vi "SR830 - Kepco - Hysteresis Measurment - Stepped DC.vi"() -> ()   [LabVIEW 2016]
uses:
  <vilib>/express/express shared/transition.llb/Dynamic To Waveform Array.vi
  <vilib>/express/express signal manip/GetorSetDDTAttributes/Set DDT Attributes/SetT0.vi
  <vilib>/express/express shared/transition.llb/Waveform Array To Dynamic.vi
  <vilib>/express/express signal manip/GetorSetDDTAttributes/Set DDT Attributes/Set DDT Properties.xnode
panel:
  out "Sample VDC (V)":dbl
  out "Over Temp":bool
  in  "Zero Field Wait Time (s)":u32=30
  out "Setup Data":T1
  in  "Sample Name":string="test"
  in  "Directory":string="D:\\JDark\\MTJ Cryostat\\test"
  out "Filename Out":path=path "D:/JDark/MTJ Cryostat/test/test-20mT-hysteresis.lvm"
  in  "Accepted Setup":bool
  in  "Verified Setup":bool
  out "Field Vs Res Noise":cluster{dbl[], dbl[]}(graph)={[-0.0544, 0.4456, 0.9352, 1.4248, 1.9143999999999999, 2.404, 2.8935999999999997, 3.3832, 3.8728, 4.362399999999999, 4.852, 5.3416, 5.8312, 6.320799999999999, 6.8104000000000005, 7.3, 7.7896, 8.2792, 8.768799999999999, 9.2584, 10.248000000000001, 10.7272, 11.216800000000001, 11.706399999999999, 12.196, 12.685599999999999, 13.1752, 13.6648, 14.154399999999999, 14.644, 15.133600000000001, 15.6232, 16.1128, 16.6024, 17.092, 17.581599999999998, 18.0712, 18.5608, 19.0504, 19.54, 20.0296, 19.519199999999998, 19.0296, 18.54, 18.0504, 17.5608, 17.0712, 16.581599999999998, 16.092, 15.6024, 15.112799999999998, 14.6232, 14.133600000000001, 13.644, 13.154399999999999, 12.6648, 12.1752, 11.685599999999999, 11.196, 10.706399999999999, 10.216800000000001, 9.7272, 9.237599999999999, 8.748000000000001, 7.7584, 7.2791999999999994, 6.7896, 6.3, 5.8104000000000005, 5.320799999999999, 4.8312, 4.3416, 3.8520000000000003, 3.3623999999999996, 2.8728, 2.3832, 1.8935999999999997, 1.4040000000000001, 0.9143999999999999, 0.42480000000000007, -0.06480000000000002, -0.5544, -1.044, -1.5335999999999999, -2.0232, -2.5128, -3.0023999999999997, -3.492, -3.9816, -4.4712, -4.9608, -5.4504, -5.94, -6.4296, -6.919199999999999, -7.4088, -7.8984000000000005, -8.387999999999998, -8.8776, -9.3672, -9.8568, -10.3464, -10.836, -11.3256, -11.815199999999999, -12.3048, -12.7944, -13.283999999999999, -13.7736, -14.2632, -14.7528, -15.7424, -16.2216, -16.711199999999998, -17.2008, -17.6904, -18.18, -18.6696, -19.159200000000002, -19.648799999999998, -20.138399999999997, -19.628, -19.138399999999997, -18.648799999999998, -18.159200000000002, -17.6696, -17.18, -16.6904, -16.2008, -15.711199999999998, -15.221599999999999, -14.732000000000001, -14.2424, -13.2528, -12.7736, -12.283999999999999, -11.7944, -11.3048, -10.815199999999999, -10.3256, -9.836, -9.3464, -8.8568, -8.3672, -7.877599999999999, -7.387999999999999, -6.8984000000000005, -6.4088, -5.919199999999999, -5.4296, -4.94, -4.4504, -3.9608, -3.4711999999999996, -2.9816, -2.492, -2.0023999999999997, -1.5128, -1.0231999999999999, -0.5335999999999999, -0.04400000000000004], [15446.997899211381, 33956.24923800761, 28583.62141204098, 32537.69937438095, 21226.11553919723, 21221.33942488045, 39173.4048903721, 26230.601252371347, 25250.361708040735, 35822.515248200485, 37581.515773031526, 23883.174686296858, 39995.65587105874, 17569.924451207833, 34863.32464679369, 18416.192176577308, 23302.25342512084, 32855.534688062005, 48354.66753159789, 26888.48894404787, 27946.841353229545, 28447.25655247211, 22692.535929595357, 30888.946076662316, 42324.47121995423, 35843.85501529699, 36799.549654445036, 33329.48011847423, 22851.300082707552, 41191.92793475303, 34456.720236005174, 26058.631203020544, 44746.53461020991, 37224.99718726645, 68825.00201996259, 42958.99230679308, 40714.67079910066, 57747.71988536508, 29691.254129653025, 64211.258772769135, 19160.606846375562, 46321.221303721766, 71029.59431320045, 46892.27695542654, 44799.75730671692, 66819.48067982277, 33651.5376743769, 59810.240340936194, 40119.21014462293, 32334.725091976245, 28529.285706498602, 23730.97499127908, 57610.91864749145, 22435.444676456966, 40951.30401185154, 25070.447710137123, 41949.69263686712, 45718.11923108557, 65627.3156788876, 56953.651543237196, 32173.835671959445, 52671.5915678221, 19668.458783462793, 66303.20158982599, 29710.854540049048, 31775.497941348356, 40549.964623149535, 51075.99354753492, 30654.539201948188, 39128.479352554976, 76442.95433228796, 39447.51980352633, 50016.20330851342, 31887.563882788363, 51028.591960972844, 10819.279889052948, 33818.527611194106, 28613.771934449134, 26922.398338747033, 48873.51208949818, 15542.950456565659, 36990.502142052654, 43527.933077723064, 44359.638776024505, 57036.44671814811, 39849.33042216752, 41185.472573773004, 39269.88832369224, 38812.156278821516, 34044.05435458031, 46110.809967419984, 26920.93030568665, 20022.36039942582, 30293.79168452148, 36986.91194556142, 31863.995532675028, 48564.8883204678, 31712.338377027238, 27426.89264464971, 30851.999129154938, 48273.56430512302, 29150.41172792822, 24567.903850798903, 63596.70014848106, 48763.27199117811, 37803.08487296523, 25487.82251127746, 36390.95236019352, 40160.54536019719, 34535.106643400075, 21909.398015546907, 27598.43480264338, 35167.06869216419, 21013.991394512836, 34624.77760643399, 30213.396643427317, 37149.78361918999, 43845.320556022314, 42048.2311943678, 27051.29365915422, 64603.25813602039, 43018.44966767505, 55993.00123154771, 50035.68025960878, 39493.42322008669, 32009.408479252674, 26595.55919730376, 42173.5517388975, 12637.40264403457, 39752.76755871613, 63107.71184796988, 40876.126484711815, 20174.17913949147, 42100.458189798745, 40400.4870213476, 24357.325777515885, 31546.25760360981, 54921.53998993925, 23599.30892344478, 34629.83814368073, 29691.38924623618, 41182.45982586981, 37153.31598804947, 14587.365677128682, 41348.93298571064, 10205.174478406218, 44091.93656368952, 31245.442862556854, 43901.36431959185, 32472.003090461087, 69163.31002984302, 21452.1832368206, 22799.206544846253, 35507.71909151544, 49297.22538812266, 29873.140517007283, 32041.329961389703, 53622.65124570277, 26624.64715323181, 29899.602878098507, 50511.70265602952]}
  out "TMR":cluster{dbl[], dbl[]}(graph)={[-0.0544, 0.4456, 0.9352, 1.4248, 1.9143999999999999, 2.404, 2.8935999999999997, 3.3832, 3.8728, 4.362399999999999, 4.852, 5.3416, 5.8312, 6.320799999999999, 6.8104000000000005, 7.3, 7.7896, 8.2792, 8.768799999999999, 9.2584, 10.248000000000001, 10.7272, 11.216800000000001, 11.706399999999999, 12.196, 12.685599999999999, 13.1752, 13.6648, 14.154399999999999, 14.644, 15.133600000000001, 15.6232, 16.1128, 16.6024, 17.092, 17.581599999999998, 18.0712, 18.5608, 19.0504, 19.54, 20.0296, 19.519199999999998, 19.0296, 18.54, 18.0504, 17.5608, 17.0712, 16.581599999999998, 16.092, 15.6024, 15.112799999999998, 14.6232, 14.133600000000001, 13.644, 13.154399999999999, 12.6648, 12.1752, 11.685599999999999, 11.196, 10.706399999999999, 10.216800000000001, 9.7272, 9.237599999999999, 8.748000000000001, 7.7584, 7.2791999999999994, 6.7896, 6.3, 5.8104000000000005, 5.320799999999999, 4.8312, 4.3416, 3.8520000000000003, 3.3623999999999996, 2.8728, 2.3832, 1.8935999999999997, 1.4040000000000001, 0.9143999999999999, 0.42480000000000007, -0.06480000000000002, -0.5544, -1.044, -1.5335999999999999, -2.0232, -2.5128, -3.0023999999999997, -3.492, -3.9816, -4.4712, -4.9608, -5.4504, -5.94, -6.4296, -6.919199999999999, -7.4088, -7.8984000000000005, -8.387999999999998, -8.8776, -9.3672, -9.8568, -10.3464, -10.836, -11.3256, -11.815199999999999, -12.3048, -12.7944, -13.283999999999999, -13.7736, -14.2632, -14.7528, -15.7424, -16.2216, -16.711199999999998, -17.2008, -17.6904, -18.18, -18.6696, -19.159200000000002, -19.648799999999998, -20.138399999999997, -19.628, -19.138399999999997, -18.648799999999998, -18.159200000000002, -17.6696, -17.18, -16.6904, -16.2008, -15.711199999999998, -15.221599999999999, -14.732000000000001, -14.2424, -13.2528, -12.7736, -12.283999999999999, -11.7944, -11.3048, -10.815199999999999, -10.3256, -9.836, -9.3464, -8.8568, -8.3672, -7.877599999999999, -7.387999999999999, -6.8984000000000005, -6.4088, -5.919199999999999, -5.4296, -4.94, -4.4504, -3.9608, -3.4711999999999996, -2.9816, -2.492, -2.0023999999999997, -1.5128, -1.0231999999999999, -0.5335999999999999, -0.04400000000000004], [69953790.21982746, 69994462.77777442, 69967718.61112727, 69943886.0679804, 69954151.73827492, 69916400.47914164, 69966503.45277163, 70017098.40182951, 69957853.90222359, 69979684.38822944, 69966894.03478292, 69958273.31269251, 69970597.54758538, 69927091.5685481, 69951274.15493505, 69975111.73394063, 70025342.38913666, 70101179.50987609, 69983374.78232008, 69890957.2826106, 69969758.43611526, 69983374.78232008, 70010101.95320812, 70010550.95864438, 69965649.97392254, 70003932.33277875, 70017895.18756127, 69996084.29346387, 69998589.10374463, 69964854.37679826, 69973057.12818795, 69978454.34335361, 69973491.18977337, 69934851.8795055, 69940590.12561432, 69990307.98671071, 69945129.35499595, 69997734.84194495, 69927452.81109615, 69944305.31098829, 69948411.266759, 69959922.07844894, 69958287.77521215, 70005177.75540388, 69971827.3162728, 69998965.56471586, 70030675.21091811, 69935227.65522334, 69997343.9155331, 69980494.7943649, 69945519.69840819, 70003917.85138094, 69957029.55837137, 70012593.28185017, 70001847.07317972, 69909770.75678013, 69937308.9477036, 69987876.14275324, 69924981.98660928, 69987470.85185637, 69960732.02693424, 69978816.11676958, 69972666.47736529, 69924187.31409012, 69952965.97173885, 69972246.8943031, 69939332.5452715, 69942238.05796859, 69858941.36052282, 69882355.26151025, 70024096.2489493, 70124276.56048097, 69971451.1471442, 69939361.45465657, 69920922.12205227, 69889687.05228348, 69905712.65829201, 69917585.00637151, 70006408.7399148, 70001065.13285743, 69964839.91156349, 69978816.11676958, 69981276.27520046, 69989511.82871358, 69995693.38548763, 69987051.09123293, 69991567.40089324, 69934447.20247924, 69914334.87523946, 69930328.43488088, 69991147.59112982, 69944666.73140821, 70003541.33714098, 69925791.1262778, 69958663.8028221, 69971017.11086768, 69906940.14727889, 69948396.80832255, 69947977.51626554, 69937323.40155673, 69999834.3362578, 69952503.24448285, 69969787.37065852, 69987847.19324781, 69996504.16244982, 69969006.1463901, 69999805.37685895, 69945910.04617715, 69983780.02577896, 69952069.44324002, 69915114.8791537, 69902376.9942027, 69955380.92894632, 69934447.20247924, 69907330.06456648, 69929114.57489035, 69894190.80452518, 69869557.18013413, 69849539.82325777, 69800352.8141219, 69815113.16441435, 69904066.44661842, 69830254.40704262, 69854398.89081328, 69919246.30120051, 69819607.31039546, 69818339.67217934, 69888445.73543541, 69870004.38464876, 69904860.66186896, 69950912.66622883, 69949192.0312033, 69964839.91156349, 69961165.93562299, 69973057.12818795, 69985415.52028471, 69938118.3726788, 69967328.01990989, 69967284.62115493, 69976775.76364617, 69951274.15493505, 69948006.43279776, 69941414.0820846, 69985429.99402861, 70005554.28724681, 69963234.3076816, 69973491.18977337, 69992826.86040007, 69995288.00404988, 69972217.95772569, 69924996.4353677, 69988715.68882897, 70001456.10083497, 69972246.8943031, 69989540.77959612, 69997387.35158546, 69967747.54398352, 69981710.43876189, 69917613.89778097, 69917628.34349464, 70040980.87136921]}
  out "Field (mT)":dbl=-0.04400000000000004
  out "Sample Resistance StDev (Ohms)":dbl=50511.70265602952
  out "Sample Resistance (Ohms)":dbl=70040980.87136921
  out "Temp StDev (K)":dbl=0.3443986882799053 format="%0.3f"
  out "Temp (K)":dbl=7.984841572107988 format="%0.3f"
  out "error out":errorcluster
  in  "Step Size (mT)":dbl=0.5 format="%#_13g"
  in  "Field Amplitude (mT)":dbl=2.0 format="%#_13g"
  in  "Rl":dbl=24060.0 format="%#_13g"
  in  "Rp":dbl=1010.0 format="%#_13g"
  in  "error in (no error)":errorcluster
  in  "VISA resource name":refnum<visa-resource-name>="SR830LockIn2"
  # "No final Slashes!"
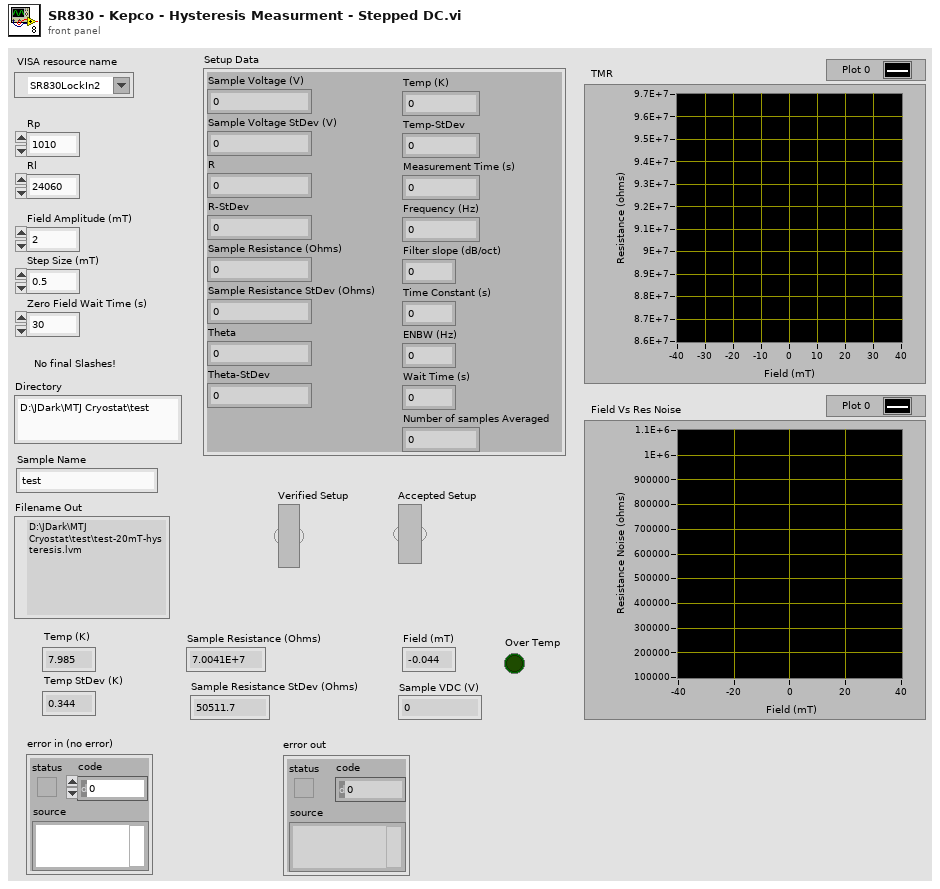
[diagram p1: front panel]
types:
  T1 = cluster{"Sample Voltage (V)":dbl, "Sample Voltage StDev (V)":dbl, "R":dbl, "R-StDev":dbl, "Sample Resistance (Ohms)":dbl, "Sample Resistance StDev (Ohms)":dbl, "Theta":dbl, "Theta-StDev":dbl, "Temp (K)":dbl, "Temp-StDev":dbl, "Measurement Time (s)":dbl, "Frequency (Hz)":dbl, "Filter slope (dB/oct)":dbl, "Time Constant (s)":dbl, "ENBW (Hz)":dbl, "Wait Time (s)":dbl, "Number of samples Averaged":dbl}
  T2 = cluster{"Sample Voltage (V)":dbl, "Sample Voltage StDev (V)":dbl, "R":dbl, "R-StDev":dbl, "Sample Resistance (Ohms)":dbl, "Sample Resistance StDev (Ohms)":dbl, "Theta":dbl, "Theta-StDev":dbl, "Temp (K)":dbl, "Temp-StDev":dbl, "Measurement Time (s)":dbl}
  T3 = cluster{"Sample Voltage (V)":dbl, "Sample Voltage StDev (V)":dbl, "R":dbl, "R-StDev":dbl, "Sample Resistance (Ohms)":dbl, "Sample Resistance StDev (Ohms)":dbl, "Theta":dbl, "Theta-StDev":dbl, "Temp (K)":dbl, "Temp-StDev":dbl, "Measurement Time (s)":dbl, "ReadOut":dbl, "Filter slope (dB/oct)":dbl, "Time Constant (s)":dbl, "ENBW":dbl, "Wait Time (s)":dbl, "Number of samples Averaged":dbl}
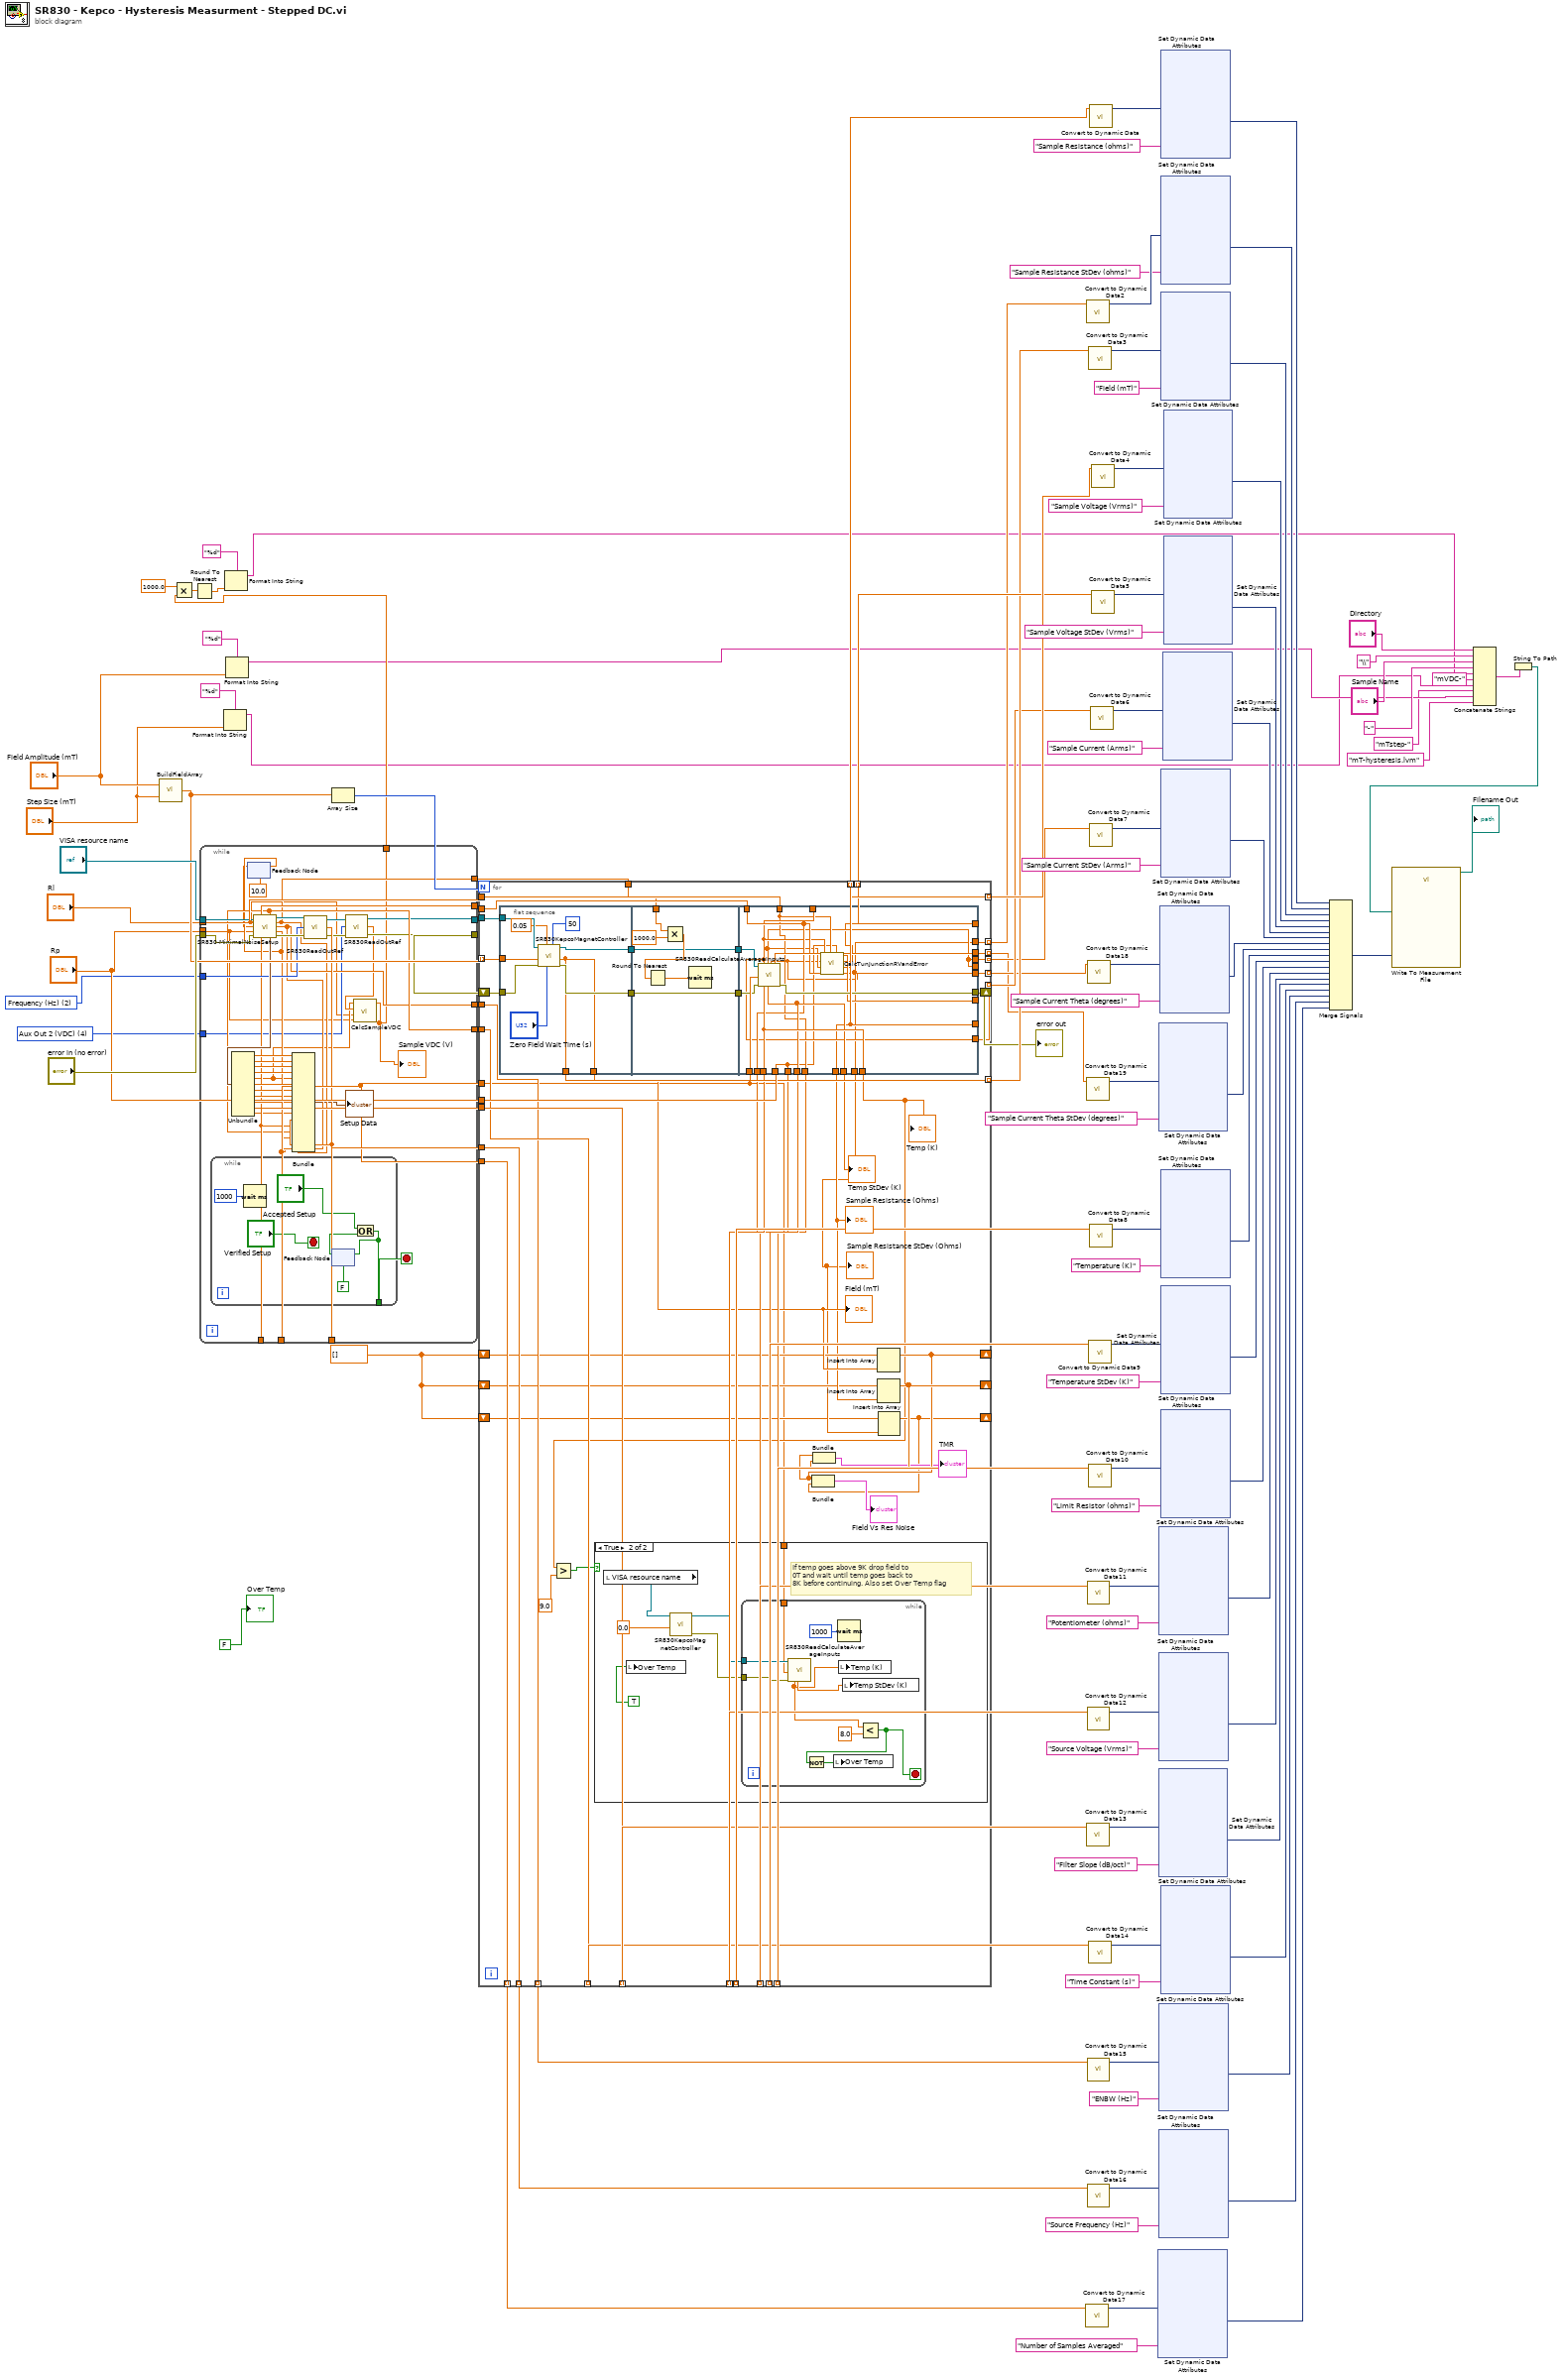
[diagram p0: block diagram]
diagram:
  w12 = u16 4 items=["Voltage Out (Vrms)"=1, "Frequency (Hz)"=2, "Aux Out 1 (VDC)"=3, "Aux Out 2 (VDC)"=4, "Time Constant (s)"=5, "Roll-Off Slope (dB/oct)"=6] ("ReadOut (1: Voltage Amplitude)")
  w25 = u16 2 items=["Voltage Out (Vrms)"=1, "Frequency (Hz)"=2, "Aux Out 1 (VDC)"=3, "Aux Out 2 (VDC)"=4, "Time Constant (s)"=5, "Roll-Off Slope (dB/oct)"=6] ("ReadOut (1: Voltage Amplitude)")
  w26 = dbl[] []
  n1 = call "BuildFieldArray.vi"("Step Size (mT)"="Step Size (mT)", "Field Amplitude (mT)"="Field Amplitude (mT)") -> ("Field Array"=w116:dbl[])
  n2 = while {
    tunnel: "Rp" -> [w121]
    tunnel: [w152] -> w114
    tunnel: "Rl" -> [w122]
    tunnel: [w138] -> w68
    tunnel: [w134] -> w66
    tunnel: [w137] -> w63
    tunnel: [w136] -> w61
    tunnel: [w139] -> w59
    tunnel: [w131] -> w47
    tunnel: "error in (no error)" -> [w155]
    tunnel: [w127] -> w27
    tunnel: "VISA resource name" -> [w156]
    tunnel: [w126] -> w48
    tunnel: w25 -> [w140]
    tunnel: w12 -> [w125]
    tunnel: [w120] -> w10
    stop <- w135 stop-if-true
    n3 = while {
      tunnel: [w157] -> w135
      stop <- "Verified Setup" stop-if-true
      n4 = Wait (ms)(milliseconds to wait=u32 1000) -> ()  [unwired: 1 out]
      n5 = feedback #1(FALSE ("Accepted Setup")) -> (w158:bool)
      n6 = Or(x="Accepted Setup", y=w158) -> (x .or. y?=w157:bool)
      n7 = feedback-in #1(w157) -> ()
    }
    n8 = feedback #2(10.0 ("Number of samples Averaged")) -> (w130:dbl)
    n9 = call "SR830-MinimalNoiseSetup.vi"("VISA resource name"=w156, "Rl"=w122, "number of averaging points"=w130, "Rp"=w121, "error in (no error)"=w155) -> ("Vs (Vrms)"=w152:dbl, "Time Constant (s)"=w137:dbl, "VISA resource name out"=w154:refnum<visa-resource-name>, "Wait Time (s)"=w134:dbl, "ENBW"=w136:dbl, "Number of samples Averaged"=w131:dbl, "Filter slope (dB/oct)"=w138:dbl, "Setup Data"=w151:T2, "error out"=w153:errorcluster)  [unwired: 2 in]
    n10 = Unbundle(w151) -> ("Sample Voltage (V)"=w150:dbl, "Sample Voltage StDev (V)"=w149:dbl, "R"=w148:dbl, "R-StDev"=w147:dbl, "Sample Resistance (Ohms)"=w123:dbl, "Sample Resistance StDev (Ohms)"=w146:dbl, "Theta"=w145:dbl, "Theta-StDev"=w144:dbl, "Temp (K)"=w143:dbl, "Temp-StDev"=w142:dbl, "Measurement Time (s)"=w141:dbl)
    n11 = feedback-in #2(w131) -> ()
    n12 = call "SR830ReadOutRef.vi"("error in (no error)"=w153, "ReadOut (1: Voltage Amplitude)"=w140, "VISA resource name"=w154) -> ("error out"=w128:errorcluster, "ReadOut"=w139:dbl, "VISA resource name out"=w129:refnum<visa-resource-name>)
    n13 = Bundle("Sample Voltage (V)"=w150, "Sample Voltage StDev (V)"=w149, "R"=w148, "R-StDev"=w147, "Sample Resistance (Ohms)"=w123, "Sample Resistance StDev (Ohms)"=w146, "Theta"=w145, "Theta-StDev"=w144, "Temp (K)"=w143, "Temp-StDev"=w142, "Measurement Time (s)"=w141, "ReadOut"=w139, "Filter slope (dB/oct)"=w138, "Time Constant (s)"=w137, "ENBW"=w136, "Wait Time (s)"=w134, "Number of samples Averaged"=w131) -> (→"Setup Data":T3)  [unwired: 1 in]
    n14 = call "SR830ReadOutRef.vi"("error in (no error)"=w128, "ReadOut (1: Voltage Amplitude)"=w125, "VISA resource name"=w129) -> ("error out"=w127:errorcluster, "ReadOut"=w124:dbl, "VISA resource name out"=w126:refnum<visa-resource-name>)
    n15 = call "CalcSampleVDC.vi"("Rp"=w121, "Rl"=w122, "VDC (V)"=w124, "Sample Resistance (Ohms)"=w123) -> ("Sample VDC (V)"=w120:dbl)  [unwired: 7 in]
    "Sample VDC (V)" <- w120
  }
  n16 = Multiply(x=1000.0, y=w10) -> (x*y=w2:dbl)
  n17 = Round To Nearest(number=w2) -> (nearest integer value=w1:dbl)
  n18 = Format Into String(format string="%d", "Step Size (mT)") -> (resulting string=w5:string)  [unwired: 2 in, 1 out]
  n19 = Format Into String(format string="%d", w1) -> (resulting string=w4:string)  [unwired: 2 in, 1 out]
  n20 = Format Into String(format string="%d", "Field Amplitude (mT)") -> (resulting string=w7:string)  [unwired: 2 in, 1 out]
  n21 = Array Size(array=w116) -> (size(s)=w117:i32)
  n22 = for {
    N: w117 -> [_]
    tunnel: w116 -> [w209] mode=indexing
    tunnel: "Rp" -> [w208]
    tunnel: "Rl" -> [w207]
    tunnel: w114 -> [w206]
    tunnel: [w205] -> w80 mode=indexing
    tunnel: [w204] -> w79 mode=indexing
    tunnel: [w203] -> w78 mode=indexing
    tunnel: [w202] -> w77 mode=indexing
    tunnel: [w201] -> w76 mode=indexing
    tunnel: [w200] -> w75 mode=indexing
    tunnel: [w199] -> w74 mode=indexing
    tunnel: [w198] -> w73 mode=indexing
    tunnel: [w197] -> w72 mode=indexing
    tunnel: [w196] -> w71 mode=indexing
    tunnel: [w195] -> w70 mode=indexing
    tunnel: [w194] -> w69 mode=indexing
    tunnel: [w193] -> w67 mode=indexing
    tunnel: w68 -> [w193]
    tunnel: w66 -> [w192]
    tunnel: w63 -> [w191]
    tunnel: [w191] -> w62 mode=indexing
    tunnel: w61 -> [w190]
    tunnel: [w190] -> w60 mode=indexing
    tunnel: w59 -> [w189]
    tunnel: [w189] -> w58 mode=indexing
    tunnel: w47 -> [w188]
    tunnel: [w188] -> w57 mode=indexing
    tunnel: w48 -> [w187]
    tunnel: w47 -> [w163]
    tunnel: [w182] -> w30 mode=indexing
    tunnel: [w181] -> w29 mode=indexing
    shift-right: [w180] -> w28
    shift-left: w27 -> [w179]
    shift-right: [w170] -> _
    shift-left: w26 -> [w176]
    shift-right: [w171] -> _
    shift-left: w26 -> [w174]
    shift-right: [w167] -> _
    shift-left: w26 -> [w172]
    n23 = flat-sequence {
      tunnel: w209 -> [w233]
      tunnel: [w227] -> w201
      tunnel: w187 -> [w231]
      tunnel: [w230] -> w185
      tunnel: [w229] -> w183
      tunnel: w179 -> [w228]
      tunnel: [w227] -> w177
      tunnel: w192 -> [w239]
      tunnel: [w235] -> w186
      tunnel: w185 -> [w235]
      tunnel: [w234] -> w184
      tunnel: w183 -> [w234]
      tunnel: [w243] -> w203
      tunnel: [w241] -> w202
      tunnel: [w244] -> w204
      tunnel: [w242] -> w205
      tunnel: [w248] -> _
      tunnel: [w245] -> _
      tunnel: w208 -> [w246]
      tunnel: w207 -> [w247]
      tunnel: w206 -> [w249]
      tunnel: [w248] -> w200
      tunnel: [w245] -> w199
      tunnel: [w251] -> w198
      tunnel: [w250] -> w197
      tunnel: [w247] -> w196
      tunnel: [w246] -> w195
      tunnel: [w249] -> w194
      tunnel: w163 -> [w256]
      tunnel: w186 -> [w255]
      tunnel: w184 -> [w254]
      tunnel: [w240] -> w182
      tunnel: [w253] -> w181
      tunnel: [w252] -> w180
      tunnel: [w251] -> w165
      tunnel: [w250] -> w178
      tunnel: [w242] -> w175
      tunnel: [w241] -> w173
      frame #0 {
        n24 = call "SR830KepcoMagnetController.vi"("Field dwell time (ms)"=u32 50, "Zero Field Wait (s)"="Zero Field Wait Time (s)", "Field Step size (mT)"=0.05, "error in (no error)"=w228, "Target Field (mT)"=w233, "VISA resource name"=w231) -> ("error out"=w230:errorcluster, "Final Field (mT)"=w227:dbl, "VISA resource name out"=w229:refnum<visa-resource-name>)  [unwired: 2 in, 1 out]
      }
      frame #1 {
        n25 = Multiply(x=w239, y=1000.0) -> (x*y=w237:dbl)
        n26 = Round To Nearest(number=w237) -> (nearest integer value=w236:dbl)
        n27 = Wait (ms)(milliseconds to wait=w236) -> ()  [unwired: 1 out]
      }
      frame #2 {
        n28 = call "SR830ReadCalculateAverageInputs.vi"("VISA resource name"=w254, "number of averaging points"=w256, "error in (no error)"=w255) -> ("R"=w248:dbl, "Temp (K)"=w251:dbl, "R-StDev"=w245:dbl, "Temp-StDev"=w250:dbl, "Theta (degrees)"=w240:dbl, "Theta-StDev (degrees)"=w253:dbl, "error out"=w252:errorcluster)  [unwired: 7 in, 3 out]
        n29 = call "CalcTunJunctionRVandError.vi"("Rp"=w246, "Rl"=w247, "Source Voltage (V)"=w249, "Sample Current StDev (A)"=w245, "Sample Current Theta (degrees)"=w240, "Sample Current R (A)"=w248) -> ("Sample Resistance StDev (Ohms)"=w241:dbl, "Sample Resistance (Ohms)"=w242:dbl, "Sample Voltage StDev (V)"=w243:dbl, "Sample Voltage (V)"=w244:dbl)  [unwired: 2 in]
      }
    }
    n30 = Greater?(x=w165, y=9.0) -> (0:w166:bool)
    n31 = case shown="True" w166 {
      tunnel: w163 -> [_ w210]
      frame False {
        # "If temp is below 9K continue as normal"
      }
      frame True {
        # "If temp goes above 9K drop field to\n0T and wait until temp goes back to\n8K before continuing. Also set Over Temp flag"
        n32 = local read "VISA resource name"() -> (w214:refnum<visa-resource-name>)
        n33 = local write "Over Temp"(TRUE ("Over Temp")) -> ()
        n34 = call "SR830KepcoMagnetController.vi"("Target Field (mT)"=0.0, "VISA resource name"=w214) -> ("error out"=w211:errorcluster, "VISA resource name out"=w212:refnum<visa-resource-name>)  [unwired: 6 in, 2 out]
        n35 = while {
          tunnel: w212 -> [w223]
          tunnel: w211 -> [w222]
          tunnel: w210 -> [w216]
          stop <- w217 stop-if-true
          n36 = call "SR830ReadCalculateAverageInputs.vi"("VISA resource name"=w223, "number of averaging points"=w216, "error in (no error)"=w222) -> ("Temp (K)"=w220:dbl, "Temp-StDev"=w221:dbl)  [unwired: 7 in, 8 out]
          n37 = Wait (ms)(milliseconds to wait=u32 1000) -> ()  [unwired: 1 out]
          n38 = local write "Temp (K)"(w220) -> ()
          n39 = local write "Temp StDev (K)"(w221) -> ()
          n40 = Less?(x=w220, y=8.0) -> (x < y?=w217:bool)
          n41 = Not(x=w217) -> (.not. x?=w218:bool)
          n42 = local write "Over Temp"(w218) -> ()
        }
      }
    }
    n43 = Insert Into Array(array=w176, new element=w177) -> (w170:dbl[])  [unwired: 1 in]
    n44 = Insert Into Array(array=w174, new element=w175) -> (w171:dbl[])  [unwired: 1 in]
    n45 = Bundle(w170, w171) -> (→"TMR":cluster{dbl[], dbl[]})  [unwired: 1 in]
    n46 = Insert Into Array(array=w172, new element=w173) -> (w167:dbl[])  [unwired: 1 in]
    n47 = Bundle(w170, w167) -> (→"Field Vs Res Noise":cluster{dbl[], dbl[]})  [unwired: 1 in]
    "Temp (K)" <- w165
    "Temp StDev (K)" <- w178
    "Sample Resistance (Ohms)" <- w175
    "Sample Resistance StDev (Ohms)" <- w173
    "Field (mT)" <- w177
  }
  "error out" <- w28
  n48 = call "Convert to Dynamic Data17"("Array"=w57) -> ("Dynamic Data Type"=w65:dynamicdata)  [unwired: 3 in]
  n49 = call "Convert to Dynamic Data2"("Array"=w77) -> ("Dynamic Data Type"=w110:dynamicdata)  [unwired: 3 in]
  n50 = call "Convert to Dynamic Data19"("Array"=w29) -> ("Dynamic Data Type"=w44:dynamicdata)  [unwired: 3 in]
  n51 = call "Convert to Dynamic Data13"("Array"=w67) -> ("Dynamic Data Type"=w88:dynamicdata)  [unwired: 3 in]
  n52 = call "Convert to Dynamic Data11"("Array"=w70) -> ("Dynamic Data Type"=w92:dynamicdata)  [unwired: 3 in]
  n53 = call "Convert to Dynamic Data12"("Array"=w69) -> ("Dynamic Data Type"=w90:dynamicdata)  [unwired: 3 in]
  n54 = call "Convert to Dynamic Data15"("Array"=w60) -> ("Dynamic Data Type"=w84:dynamicdata)  [unwired: 3 in]
  n55 = call "Convert to Dynamic Data16"("Array"=w58) -> ("Dynamic Data Type"=w82:dynamicdata)  [unwired: 3 in]
  n56 = call "Convert to Dynamic Data18"("Array"=w30) -> ("Dynamic Data Type"=w46:dynamicdata)  [unwired: 3 in]
  n57 = call "Convert to Dynamic Data3"("Array"=w76) -> ("Dynamic Data Type"=w108:dynamicdata)  [unwired: 3 in]
  n58 = call "Convert to Dynamic Data9"("Array"=w72) -> ("Dynamic Data Type"=w96:dynamicdata)  [unwired: 3 in]
  n59 = call "Convert to Dynamic Data10"("Array"=w71) -> ("Dynamic Data Type"=w94:dynamicdata)  [unwired: 3 in]
  n60 = call "Convert to Dynamic Data14"("Array"=w62) -> ("Dynamic Data Type"=w86:dynamicdata)  [unwired: 3 in]
  n61 = call "Convert to Dynamic Data"("Array"=w80) -> ("Dynamic Data Type"=w113:dynamicdata)  [unwired: 3 in]
  n62 = call "Convert to Dynamic Data7"("Array"=w74) -> ("Dynamic Data Type"=w100:dynamicdata)  [unwired: 3 in]
  n63 = call "Convert to Dynamic Data8"("Array"=w73) -> ("Dynamic Data Type"=w98:dynamicdata)  [unwired: 3 in]
  n64 = call "Convert to Dynamic Data6"("Array"=w75) -> ("Dynamic Data Type"=w102:dynamicdata)  [unwired: 3 in]
  n65 = call "Convert to Dynamic Data4"("Array"=w79) -> ("Dynamic Data Type"=w106:dynamicdata)  [unwired: 3 in]
  n66 = call "Convert to Dynamic Data5"("Array"=w78) -> ("Dynamic Data Type"=w104:dynamicdata)  [unwired: 3 in]
  n67 = xnode "Set Dynamic Data Attributes"("Signals In"=w65, "Signal Name"="Number of Samples Averaged") -> ("Signals Out"=w42:dynamicdata)  [unwired: 2 in, 1 out]
  n68 = xnode "Set Dynamic Data Attributes"("Signals In"=w44, "Signal Name"="Sample Current Theta StDev (degrees)") -> ("Signals Out"=w32:dynamicdata)  [unwired: 2 in, 1 out]
  n69 = xnode "Set Dynamic Data Attributes"("Signals In"=w88, "Signal Name"="Filter Slope (dB/oct)") -> ("Signals Out"=w38:dynamicdata)  [unwired: 2 in, 1 out]
  n70 = xnode "Set Dynamic Data Attributes"("Signals In"=w92, "Signal Name"="Potentiometer (ohms)") -> ("Signals Out"=w36:dynamicdata)  [unwired: 2 in, 1 out]
  n71 = xnode "Set Dynamic Data Attributes"("Signals In"=w90, "Signal Name"="Source Voltage (Vrms)") -> ("Signals Out"=w37:dynamicdata)  [unwired: 2 in, 1 out]
  n72 = xnode "Set Dynamic Data Attributes"("Signals In"=w84, "Signal Name"="ENBW (Hz)") -> ("Signals Out"=w40:dynamicdata)  [unwired: 2 in, 1 out]
  n73 = xnode "Set Dynamic Data Attributes"("Signals In"=w82, "Signal Name"="Source Frequency (Hz)") -> ("Signals Out"=w41:dynamicdata)  [unwired: 2 in, 1 out]
  n74 = xnode "Set Dynamic Data Attributes"("Signals In"=w46, "Signal Name"="Sample Current Theta (degrees)") -> ("Signals Out"=w31:dynamicdata)  [unwired: 2 in, 1 out]
  n75 = xnode "Set Dynamic Data Attributes"("Signals In"=w108, "Signal Name"="Field (mT)") -> ("Signals Out"=w53:dynamicdata)  [unwired: 2 in, 1 out]
  n76 = xnode "Set Dynamic Data Attributes"("Signals In"=w96, "Signal Name"="Temperature StDev (K)") -> ("Signals Out"=w34:dynamicdata)  [unwired: 2 in, 1 out]
  n77 = xnode "Set Dynamic Data Attributes"("Signals In"=w94, "Signal Name"="Limit Resistor (ohms)") -> ("Signals Out"=w35:dynamicdata)  [unwired: 2 in, 1 out]
  n78 = xnode "Set Dynamic Data Attributes"("Signals In"=w86, "Signal Name"="Time Constant (s)") -> ("Signals Out"=w39:dynamicdata)  [unwired: 2 in, 1 out]
  n79 = xnode "Set Dynamic Data Attributes"("Signals In"=w113, "Signal Name"="Sample Resistance (ohms)") -> ("Signals Out"=w55:dynamicdata)  [unwired: 2 in, 1 out]
  n80 = xnode "Set Dynamic Data Attributes"("Signals In"=w110, "Signal Name"="Sample Resistance StDev (ohms)") -> ("Signals Out"=w54:dynamicdata)  [unwired: 2 in, 1 out]
  n81 = xnode "Set Dynamic Data Attributes"("Signals In"=w100, "Signal Name"="Sample Current StDev (Arms)") -> ("Signals Out"=w49:dynamicdata)  [unwired: 2 in, 1 out]
  n82 = xnode "Set Dynamic Data Attributes"("Signals In"=w98, "Signal Name"="Temperature (K)") -> ("Signals Out"=w33:dynamicdata)  [unwired: 2 in, 1 out]
  n83 = xnode "Set Dynamic Data Attributes"("Signals In"=w102, "Signal Name"="Sample Current (Arms)") -> ("Signals Out"=w50:dynamicdata)  [unwired: 2 in, 1 out]
  n84 = xnode "Set Dynamic Data Attributes"("Signals In"=w106, "Signal Name"="Sample Voltage (Vrms)") -> ("Signals Out"=w52:dynamicdata)  [unwired: 2 in, 1 out]
  n85 = xnode "Set Dynamic Data Attributes"("Signals In"=w104, "Signal Name"="Sample Voltage StDev (Vrms)") -> ("Signals Out"=w51:dynamicdata)  [unwired: 2 in, 1 out]
  n86 = Merge Signals(w55, w54, w53, w52, w51, w50, w49, w31, w32, w33, w34, w35, w36, w37, w38, w39, w40, w41, w42) -> (w56:dynamicdata)
  n87 = Concatenate Strings("Directory", "\\" ("Sample 2"), "Sample Name", "-" ("Sample 2"), w4, "mVDC-" ("string"), w5, "mTstep-" ("Sample 2"), w7, "mT-hysteresis.lvm" ("Sample 2")) -> (w17:string)
  n88 = String To Path(string=w17) -> (path=w16:path)
  n89 = call "Write To Measurement File"("Signals"=w56, "Filename"=w16) -> ("Filename Out"=→"Filename Out":path)  [unwired: 15 in, 2 out]
  "Over Temp" <- FALSE ("Over Temp")
